vi "All stations scan config.vi"(10 "station idx":i32, 11 "configuration file path":path) -> (0 "error out":errorcluster caption="错误输出", 2 "station idx":i32, 3 "configuration file path":path, 5 "state scan config":T1)   [LabVIEW 2018]
uses:
  Crl defs/one state scans config.ctl
  Communication connection/Crl defs/scanner config.ctl
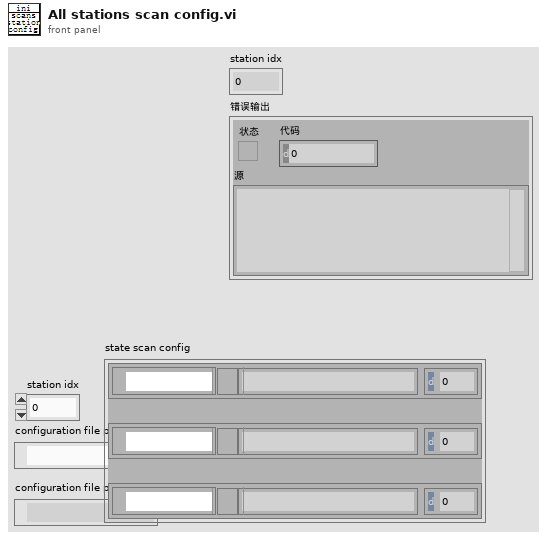
[diagram p1: front panel]
types:
  T1 = typedef "one state scans config.ctl" = cluster{"scan 1 ":T2, "scan 2":T2, "scan 3":T2}
  T2 = typedef "scanner config.ctl" = cluster{"connect ip or coms":string, "port":u16, "tcp connect id":refnum<k5>, "VISA resource name":refnum<visa-resource-name>}
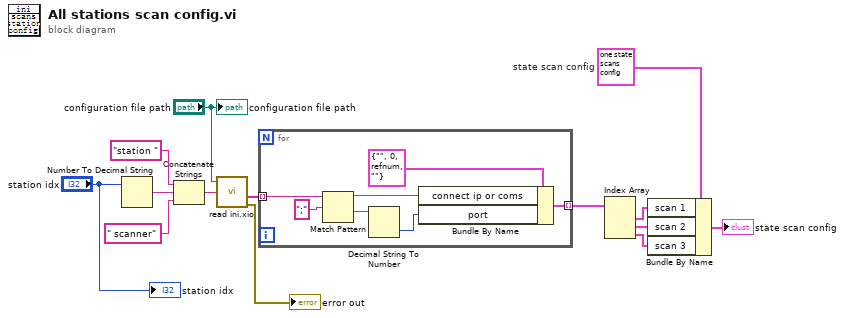
[diagram p0: block diagram]
diagram:
  w3 = T1 {"scan 1 "={"connect ip or coms"="", "port"=0, "tcp connect id"=refnum, "VISA resource name"=""}, "scan 2"={"connect ip or coms"="", "port"=0, "tcp connect id"=refnum, "VISA resource name"=""}, "scan 3"={"connect ip or coms"="", "port"=0, "tcp connect id"=refnum, "VISA resource name"=""}}  # state scan config
  n1 = Number To Decimal String(number="station idx") -> (decimal integer string=w14:string)  [unwired: 1 in]
  n2 = Concatenate Strings("station ", w14, " scanner" ("string")) -> (w11:string)
  n3 = call "read ini.xio.vi"("configuration file path"="configuration file path", "Sections"=w11) -> ("Values"=w8:string[], "error out"=→"error out":errorcluster)  [unwired: 1 in, 3 out]
  n4 = for {
    tunnel: w8 -> [w21] mode=indexing
    tunnel: [w17] -> w7 mode=indexing
    n5 = Match Pattern(string=w21, regular expression=";" ("正则表达式")) -> (before substring=w19:string, after substring=w15:string)  [unwired: 1 in, 2 out]
    n6 = Decimal String To Number(string=w15) -> (number=w18:i32)  [unwired: 2 in, 1 out]
    n7 = Bundle By Name(cluster=T2 {"connect ip or coms"="", "port"=0, "tcp connect id"=refnum, "VISA resource name"=""} ("print config"), "connect ip or coms"=w19, "port"=w18) -> (w17:T2)
  }
  n8 = Index Array(array=w7) -> (element #1=w6:T2, element #2=w5:T2, element #3=w4:T2)  [unwired: 3 in]
  n9 = Bundle By Name(cluster=w3, "scan 1"=w6, "scan 2"=w5, "scan 3"=w4) -> (→"state scan config":T1)
  "configuration file path" <- "configuration file path"
  "station idx" <- "station idx"
